vi "SetPositionPIDigital.vi"(1 "Current Position (µm)":cluster{"x":dbl, "y":dbl, "z":dbl} {"z" format="%.2f"; "y" format="%.2f"; "x" format="%.2f"}) -> (0 "error out":errorcluster)   [LabVIEW 2009]
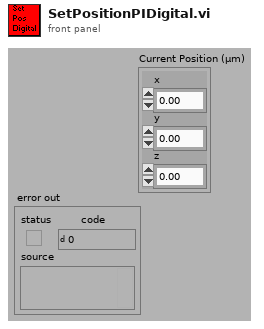
[diagram p1: front panel]
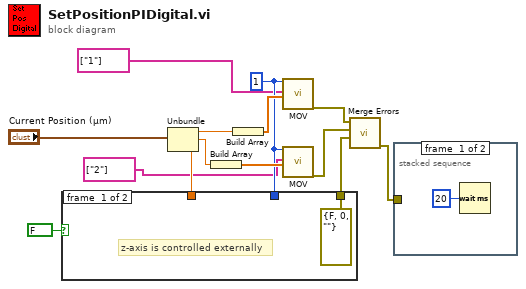
[diagram p0: block diagram]
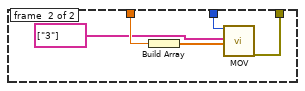
[diagram p2: hidden frame]
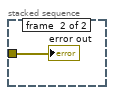
[diagram p3: hidden frame]
diagram:
  w9 = 1 ("System no.")
  n1 = Unbundle("Current Position (µm)") -> ("x"=w14:dbl, "y"=w12:dbl, "z"=w11:dbl)
  n2 = case shown="False" FALSE {
    tunnel: w11 -> [_ w20]
    tunnel: w9 -> [_ w18]
    tunnel: [errorcluster {"status"=FALSE, "code"=0, "source"=""} ("error out") w16] -> w3
    frame #0 {
      # "z-axis is controlled externally"
    }
    frame #1 {
      n3 = Build Array(w20) -> (w19:dbl[])
      n4 = call "MOV.vi"("System no."=w18, "Axes to move"=string[] ["3"], "Position values"=w19) -> ("error out"=w16:errorcluster)  [unwired: 16 in]
    }
  }
  n5 = Build Array(w12) -> (w10:dbl[])
  n6 = Build Array(w14) -> (w13:dbl[])
  n7 = call "MOV.vi"("System no."=w9, "Axes to move"=string[] ["1"], "Position values"=w13) -> ("error out"=w5:errorcluster)  [unwired: 16 in]
  n8 = call "MOV.vi"("System no."=w9, "Axes to move"=string[] ["2"], "Position values"=w10) -> ("error out"=w4:errorcluster)  [unwired: 16 in]
  n9 = call <vilib>:"Merge Errors.vi"("error in 3 (no error)"=w3, "error in 2 (no error)"=w4, "error in 1 (no error)"=w5) -> ("error out"=w2:errorcluster)  [unwired: 4 in]
  n10 = stacked-sequence {
    tunnel: w2 -> [_ w22]
    frame #0 {
      n11 = Wait (ms)(milliseconds to wait=u32 20) -> ()  [unwired: 1 out]
    }
    frame #1 {
      "error out" <- w22
    }
  }
